vi "EXA_Set_Reference_Level_Y_ACPR_Mod.vi"(0 "VISA resource name":refnum<visa-resource-name>, 9 "Reference Level \nOffset (dBm)":dbl, 11 "error in":errorcluster) -> (4 "VISA resource name":refnum<visa-resource-name>, 15 "error out":errorcluster)   [LabVIEW 2016]
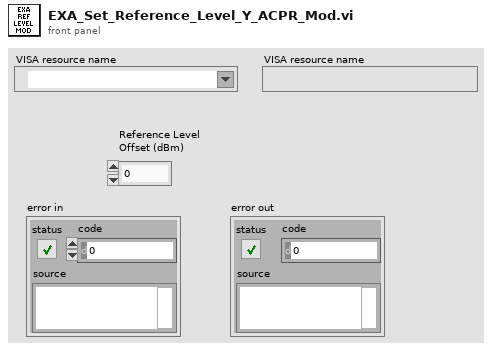
[diagram p1: front panel]
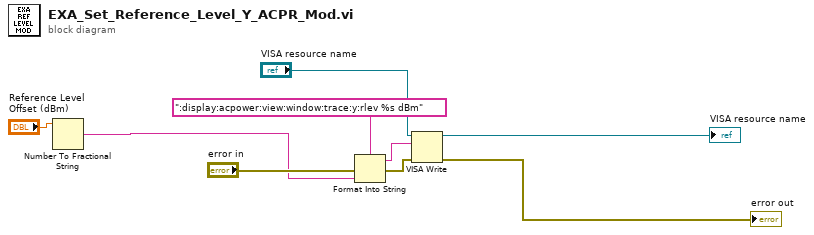
[diagram p0: block diagram]
diagram:
  n1 = Number To Fractional String(number="Reference Level \nOffset (dBm)") -> (F-format string=w1:string)  [unwired: 3 in]
  n2 = Format Into String(format string=":display:acpower:view:window:trace:y:rlev %s dBm", error in="error in", w1) -> (resulting string=w6:string, error out=w8:errorcluster)  [unwired: 1 in]
  n3 = VISA Write(VISA resource name="VISA resource name", write buffer=w6, error in (no error)=w8) -> (VISA resource name out=→"VISA resource name":refnum<visa-resource-name>, error out=→"error out":errorcluster)  [unwired: 1 out]
